vi "logStarData.vi"(8 "commandString":string, 11 "Filename":path=path "D:/googleDrive/remoteWork/builds/starSystem/starLogFile.txt") -> ()   [LabVIEW 2021]
uses:
  <vilib>/Utility/file.llb/Write Delimited Spreadsheet (string).vi
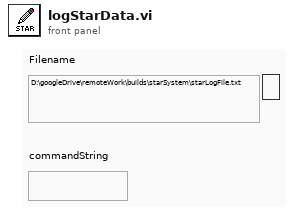
[diagram p1: front panel]
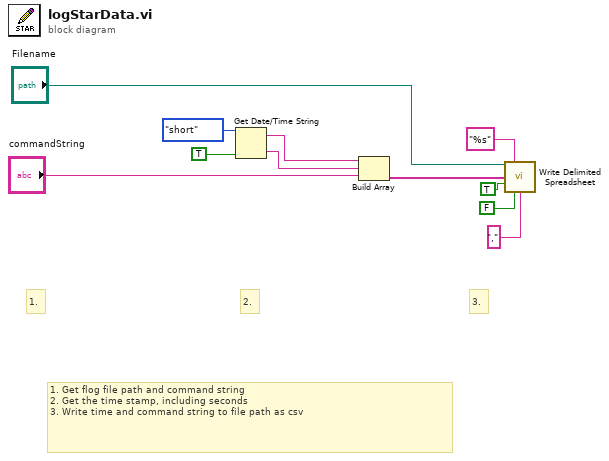
[diagram p0: block diagram]
diagram:
  # "1. Get flog file path and command string\n2. Get the time stamp, including seconds\n3. Write time and command string to file path as csv"
  # "3."
  # "1."
  # "2."
  n1 = Get Date/Time String(date format (0)=enum16{"short", "long", "abbreviated"}."short", want seconds? (F)=TRUE) -> (date string=w2:string, time string=w3:string)  [unwired: 1 in]
  n2 = Build Array(w2, w3, "commandString") -> (w4:string[])
  n3 = call-poly <vilib>:"Write Delimited Spreadsheet.vi"("file path (dialog if empty)"="Filename", "format (%s)"="%s" ("format (%.3f)"), "1D data"=w4, "append to file? (new file:F)"=TRUE, "transpose? (no:F)"=FALSE, "delimiter (\\t)"="," ("delimiter (\\t)")) -> ()  [unwired: 8 in, 2 out]
